vi "Load Settings from XML.vi"(8 "error in (no error)":errorcluster, 11 "Settings in":T1={"Hardware Configuration"={"Tasks Array"=[]}, "Logging Configuration"={"Log File Base Path"=path ""}, "Feed Module Configuration"={"Cycle Period"=0.0, "Ismatech"={"VISA resource name"="", "Simulated?"=FALSE, "Pump Number"=1.0, "Reverse?"=FALSE}, "Masterflex"={"VISA resource name"="", "Simulated?"=FALSE, "Pump Number"=1.0, "Reverse?"=FALSE}, "Mettler"={"VISA resource name"="", "Simulated?"=FALSE}, "Bronkhorst M13 Flow Meter"={"VISA resource name"="", "Simulated?"=FALSE, "Smoothing Steps"=1}, "PID 2 Parameters"={"Input Device"=enum."Flowmeter", "Output Device"=enum."Ismatec ISM 831C", "Setpoint"=0.0, "PID gains"={"proportional gain (Kc)"=1.0, "integral time (Ti, min)"=0.01, "derivative time (Td, min)"=0.0}}, "Manual Entry"=0.0, "Auto?"=TRUE, "VICI Settings"={"VISA resource name"="", "Simulated?"=FALSE, "Pump Number"=0.0, "Reverse?"=FALSE}, "output range"={"output high"=100.0, "output low"=0.0}}, "Load Count"=0.0, "TT Configuration In"={"physical channels"="cDAQ2Mod4/ai0", "name to assign"="Temp1", "units"=10143}, "PT Configuration"={"physical channels"="cDAQ2Mod8/ai15", "name to assign"="Pressure", "units"=10342}} {"PT Configuration"."units" items=["Amps"=10342, "From Custom Scale"=10065]; "TT Configuration In"."units" items=["Deg C"=10143, "Deg F"=10144, "Kelvins"=10325, "Deg R"=10145, "From Custom Scale"=10065]; "Feed Module Configuration"."output range"."output low" min=0.0 max=100.0 format="%.2f"; "Feed Module Configuration"."output range"."output high" format="%.2f"; "Feed Module Configuration"."VICI Settings"."Pump Number" min=1.0 max=20.0 step=1.0; "Feed Module Configuration"."PID 2 Parameters"."PID gains"."derivative time (Td, min)" format="%.3f"; "Feed Module Configuration"."PID 2 Parameters"."PID gains"."integral time (Ti, min)" format="%.3f"; "Feed Module Configuration"."PID 2 Parameters"."PID gains"."proportional gain (Kc)" format="%.3f"; "Feed Module Configuration"."Bronkhorst M13 Flow Meter"."Smoothing Steps" min=1 step=1; "Feed Module Configuration"."Masterflex"."Pump Number" min=1.0 max=20.0 step=1.0; "Feed Module Configuration"."Ismatech"."Pump Number" min=1.0 max=20.0 step=1.0}) -> (0 "error out":errorcluster, 3 "Settings out":T1={"Hardware Configuration"={"Tasks Array"=[]}, "Logging Configuration"={"Log File Base Path"=path ""}, "Feed Module Configuration"={"Cycle Period"=0.0, "Ismatech"={"VISA resource name"="", "Simulated?"=FALSE, "Pump Number"=1.0, "Reverse?"=FALSE}, "Masterflex"={"VISA resource name"="", "Simulated?"=FALSE, "Pump Number"=1.0, "Reverse?"=FALSE}, "Mettler"={"VISA resource name"="", "Simulated?"=FALSE}, "Bronkhorst M13 Flow Meter"={"VISA resource name"="", "Simulated?"=FALSE, "Smoothing Steps"=1}, "PID 2 Parameters"={"Input Device"=enum."Flowmeter", "Output Device"=enum."Ismatec ISM 831C", "Setpoint"=0.0, "PID gains"={"proportional gain (Kc)"=1.0, "integral time (Ti, min)"=0.01, "derivative time (Td, min)"=0.0}}, "Manual Entry"=0.0, "Auto?"=TRUE, "VICI Settings"={"VISA resource name"="", "Simulated?"=FALSE, "Pump Number"=0.0, "Reverse?"=FALSE}, "output range"={"output high"=100.0, "output low"=0.0}}, "Load Count"=0.0, "TT Configuration In"={"physical channels"="cDAQ2Mod4/ai0", "name to assign"="Temp1", "units"=10143}, "PT Configuration"={"physical channels"="cDAQ2Mod8/ai15", "name to assign"="Pressure", "units"=10342}} {"PT Configuration"."units" items=["Amps"=10342, "From Custom Scale"=10065]; "TT Configuration In"."units" items=["Deg C"=10143, "Deg F"=10144, "Kelvins"=10325, "Deg R"=10145, "From Custom Scale"=10065]; "Feed Module Configuration"."output range"."output low" min=0.0 max=100.0 format="%.2f"; "Feed Module Configuration"."output range"."output high" format="%.2f"; "Feed Module Configuration"."VICI Settings"."Pump Number" min=1.0 max=20.0 step=1.0; "Feed Module Configuration"."PID 2 Parameters"."PID gains"."derivative time (Td, min)" format="%.3f"; "Feed Module Configuration"."PID 2 Parameters"."PID gains"."integral time (Ti, min)" format="%.3f"; "Feed Module Configuration"."PID 2 Parameters"."PID gains"."proportional gain (Kc)" format="%.3f"; "Feed Module Configuration"."Bronkhorst M13 Flow Meter"."Smoothing Steps" min=1 step=1; "Feed Module Configuration"."Masterflex"."Pump Number" min=1.0 max=20.0 step=1.0; "Feed Module Configuration"."Ismatech"."Pump Number" min=1.0 max=20.0 step=1.0})   [LabVIEW 2021, in "Settings.lvlib"]
uses:
  Settings.lvlib
  <vilib>/Utility/xml.llb/Read From XML File(string).vi
  <vilib>/Utility/xml.llb/Write to XML File(string).vi
  Acquisition/Hardware Configuration.ctl
  DAQ/DAQ.lvlib
  Logging/Logging Configuration.ctl
  Logging/Logging.lvlib
  Settings.ctl
  Feed Module/Controls/Feed Module Settings Cluster.ctl
  Feed Module/Feed Module.lvlib
  Ismatec ISM 831C/Controls/Ismatech Settings Cluster.ctl
  Masterflex 7550-30/Controls/Settings Cluster.ctl
  Masterflex 7550-30/Masterflex 7550-30.lvlib
  Mettler Toledo/Controls/Settings Cluster.ctl
  Mettler Toledo/Mettler Toledo.lvlib
  Bronkhorst M13 Flow Meter/Settings Cluster.ctl
  Bronkhorst M13 Flow Meter/Bronkhorst M13 Flow Meter.lvlib
  Measure Instrument/PID Input Enum.ctl
  Measure Instrument/PID 2 Output Enum.ctl
  Measure Instrument/PID 2 Parameters Cluster.ctl
  Pressure Sensor/PT Configuration.ctl
  Pressure Sensor/Pressure.lvlib
  Acquisition/Task Cluster.ctl
  VICI M50/VICI Settings.ctl
panel:
  # "(Scroll up for Settings Controls)"
  # "Output Instruments"
  # "Input Instruments"
  # "Output Instruments"
  # "Input Instruments"
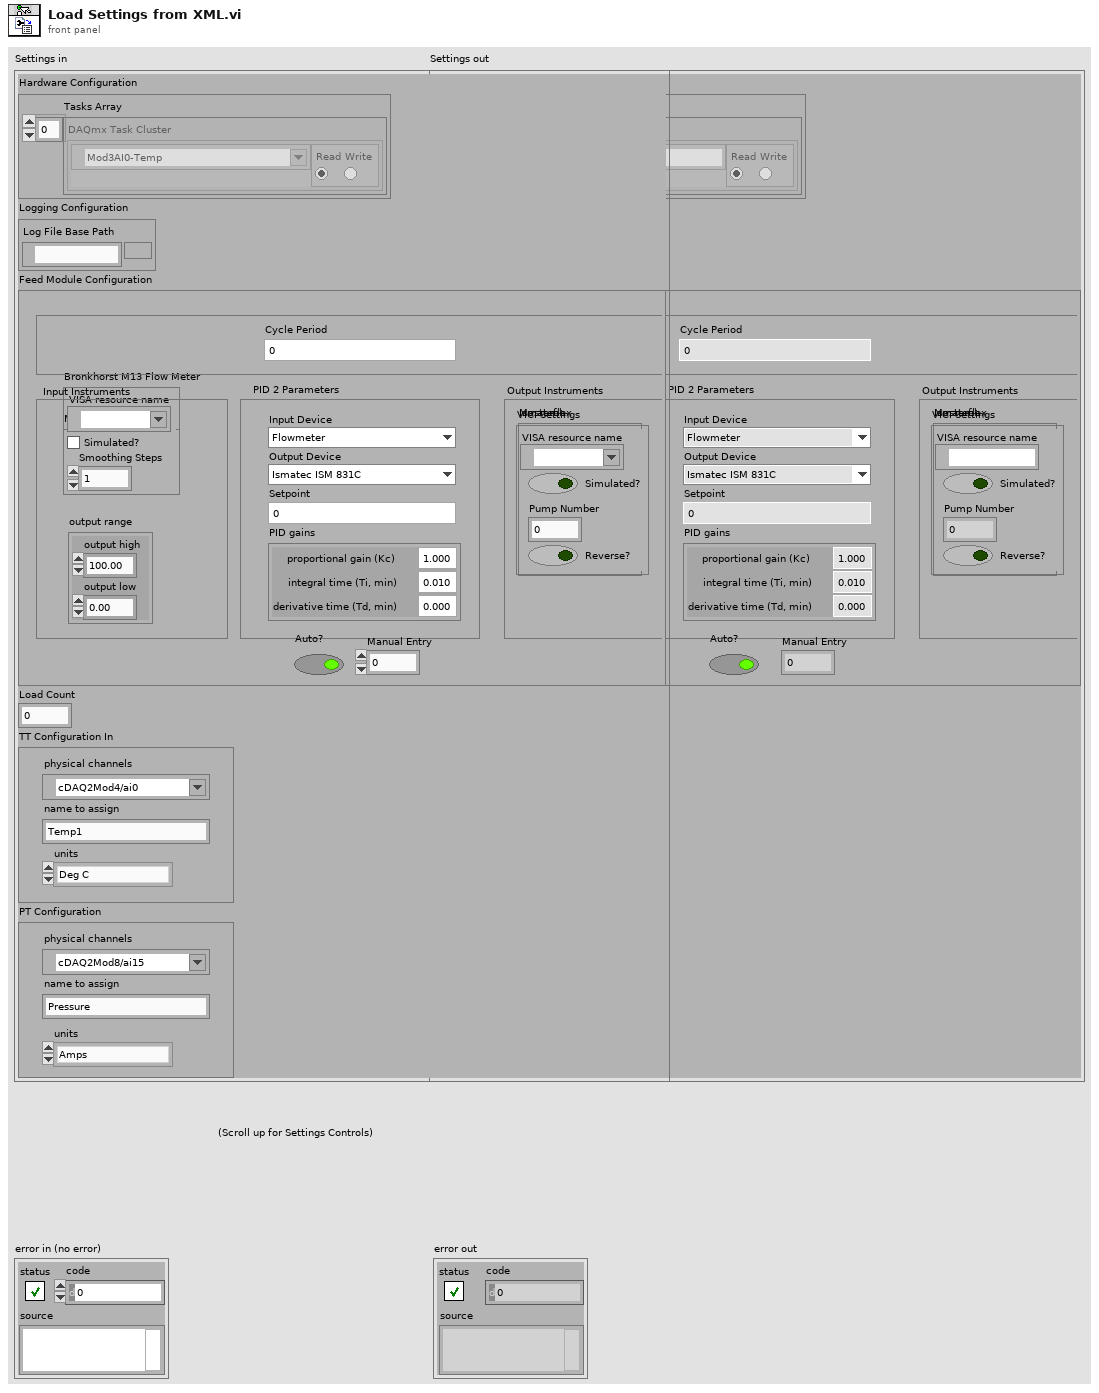
[diagram p1: front panel]
types:
  T1 = typedef "Settings.lvlib/Settings.ctl" = cluster{"Hardware Configuration":T2, "Logging Configuration":T4, "Feed Module Configuration":T5, "Load Count":dbl, "TT Configuration In":cluster{"physical channels":tag, "name to assign":string, "units":i32}, "PT Configuration":T14}
  T2 = typedef "DAQ.lvlib/Hardware Configuration.ctl" = cluster{"Tasks Array":T3[]}
  T3 = typedef "Task Cluster.ctl" = cluster{"DAQmx Task":refnum<k21>, "Read-Write Radio":enum32{"Read", "Write"}}
  T4 = typedef "Logging.lvlib/Logging Configuration.ctl" = cluster{"Log File Base Path":path}
  T5 = typedef "Feed Module.lvlib/Feed Module Settings Cluster.ctl" = cluster{"Cycle Period":dbl, "Ismatech":T6, "Masterflex":T7, "Mettler":T8, "Bronkhorst M13 Flow Meter":T9, "PID 2 Parameters":T10, "Manual Entry":dbl, "Auto?":bool, "VICI Settings":T13, "output range":cluster{"output high":dbl, "output low":dbl}}
  T6 = typedef "Ismatec ISM 831C.lvlib/Ismatech Settings Cluster.ctl" = cluster{"VISA resource name":refnum<visa-resource-name>, "Simulated?":bool, "Pump Number":dbl, "Reverse?":bool}
  T7 = typedef "Masterflex 7550-30.lvlib/Settings Cluster.ctl" = cluster{"VISA resource name":refnum<visa-resource-name>, "Simulated?":bool, "Pump Number":dbl, "Reverse?":bool}
  T8 = typedef "Mettler Toledo.lvlib/Settings Cluster.ctl" = cluster{"VISA resource name":refnum<visa-resource-name>, "Simulated?":bool}
  T9 = typedef "Bronkhorst M13 Flow Meter.lvlib/Settings Cluster.ctl" = cluster{"VISA resource name":refnum<visa-resource-name>, "Simulated?":bool, "Smoothing Steps":i32}
  T10 = typedef "PID 2 Parameters Cluster.ctl" = cluster{"Input Device":T11, "Output Device":T12, "Setpoint":dbl, "PID gains":cluster{"proportional gain (Kc)":dbl, "integral time (Ti, min)":dbl, "derivative time (Td, min)":dbl}}
  T11 = typedef "PID Input Enum.ctl" = enum16{"Default", "Flowmeter", "Scale Rate of Change"}
  T12 = typedef "PID 2 Output Enum.ctl" = enum16{"Default", "Ismatec ISM 4308", "Ismatec ISM 831C", "Masterflex 7550-30", "VICI M6", "VICI M50", "Tacmina QI", "KNF SIMDOS", "ASIA Type C", "FLOM UI-22-11", "SSI PR/LD", "SSI P40", "Masterflex 75211-70"}
  T13 = typedef "VICI Settings.ctl" = cluster{"VISA resource name":refnum<visa-resource-name>, "Simulated?":bool, "Pump Number":dbl, "Reverse?":bool}
  T14 = typedef "Pressure.lvlib/PT Configuration.ctl" = cluster{"physical channels":tag, "name to assign":string, "units":i32}
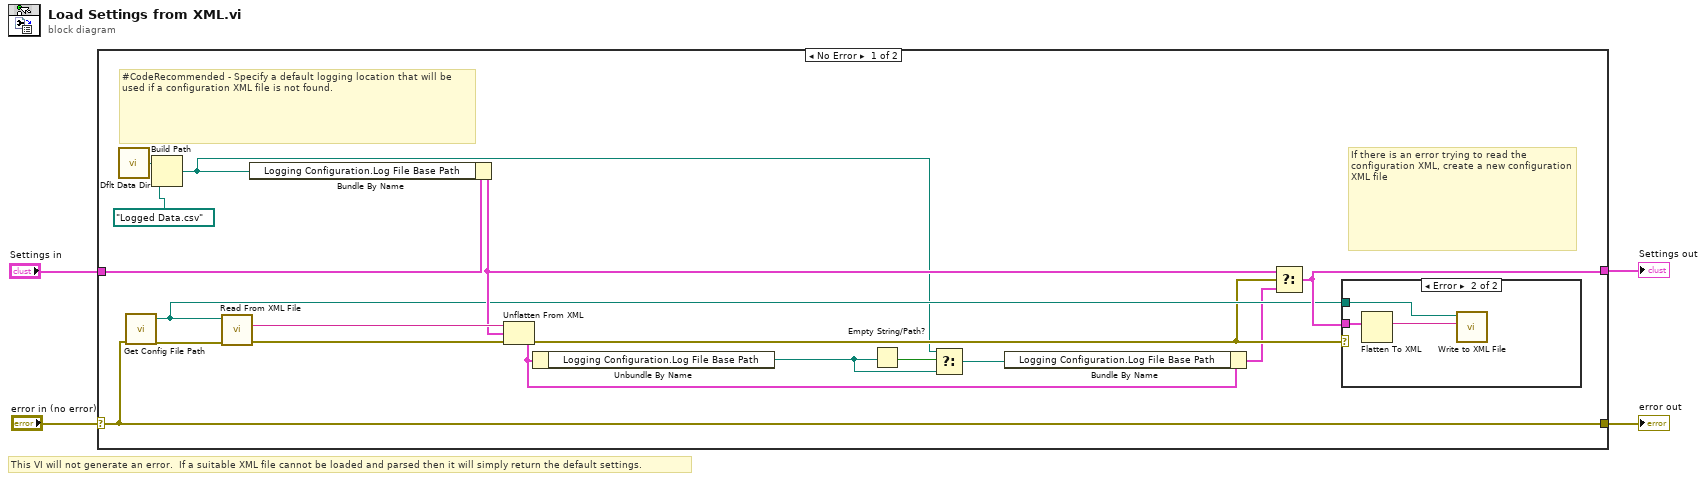
[diagram p0: block diagram]
diagram:
  # "This VI will not generate an error.  If a suitable XML file cannot be loaded and parsed then it will simply return the default settings."
  n1 = case shown="No Error" "error in (no error)" {
    selector: "error in (no error)" -> [w19 w26]
    tunnel: [w19 w26] -> w3
    tunnel: "Settings in" -> [w18 w25]
    tunnel: [w14 w25] -> w1
    frame No Error {
      # "If there is an error trying to read the configuration XML, create a new configuration XML file"
      # "#CodeRecommended - Specify a default logging location that will be used if a configuration XML file is not found."
      n2 = call <vilib>:"Dflt Data Dir.vi"() -> ("App:Default Data Directory"=w16:path)
      n3 = call "Get Config File Path.vi"("error in (no error)"=w19) -> ("error out"=w21:errorcluster, "XML File Path"=w13:path)  [unwired: 9 in]
      n4 = Build Path(base path=w16, name or relative path=path "Logged Data.csv" ("App:Default Data Directory")) -> (appended path=w9:path)
      n5 = call-poly <vilib>:"Read From XML File.vi"("error in (no error)"=w21, "XML File Path"=w13) -> ("error out"=w12:errorcluster, "XML Elements"=w20:string)  [unwired: 7 in, 1 out]
      n6 = Bundle By Name(cluster=w18, "Logging Configuration.Log File Base Path"=w9) -> (w17:T1)
      n7 = Unflatten From XML(xml string=w20, type=w17, error in (no error)=w12) -> (value=w7:T1, error out=w11:errorcluster)
      n8 = Unbundle By Name(w7) -> ("Logging Configuration.Log File Base Path"=w5:path)
      n9 = Empty String/Path?(string/path=w5) -> (empty?=w10:bool)
      n10 = Select(t=w9, s=w10, f=w5) -> (s? t:f=w8:path)
      n11 = Bundle By Name(cluster=w7, "Logging Configuration.Log File Base Path"=w8) -> (w6:T1)
      n12 = Select(t=w17, s=w11, f=w6) -> (s? t:f=w14:T1)
      n13 = case shown="Error" w11 {
        tunnel: w14 -> [_ w24]
        tunnel: w13 -> [_ w22]
        frame No Error {
        }
        frame Error {
          n14 = Flatten To XML(6:w24) -> (2:w23:string)
          n15 = call-poly <vilib>:"Write to XML File.vi"("XML Input"=w23, "XML File Path"=w22) -> ()  [unwired: 7 in, 3 out]
        }
      }
    }
    frame Error {
    }
  }
  "error out" <- w3
  "Settings out" <- w1
